vi "Create Review Test.vi"() -> ()   [LabVIEW 2018, in "Collaborator.lvlib"]
uses:
  Collaborator.lvlib
  Command Configuration.ctl
  Web Client/Web Client.lvclass
  <vilib>/JDP Science/JSONtext/JSONtext.lvlib
panel:
  out "error out":errorcluster
  out "Response":string
  in  "Address":string
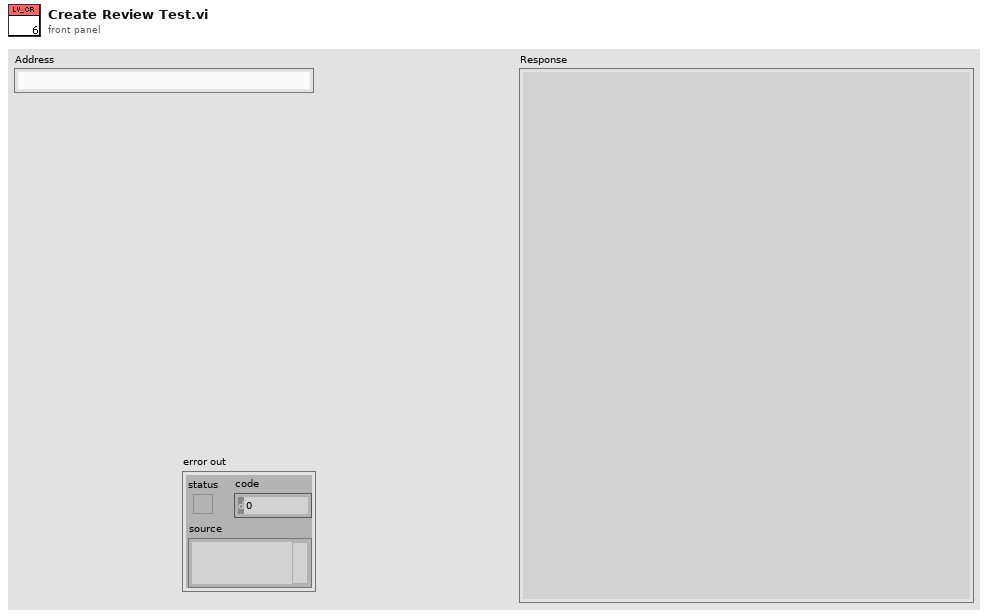
[diagram p1: front panel]
types:
  T1 = typedef "Collaborator.lvlib/Command Configuration.ctl" = cluster{"Interface Name":string, "Method Name":string, "Arguments":cluster{"Argument Name":string, "Argument Value":string}[]}
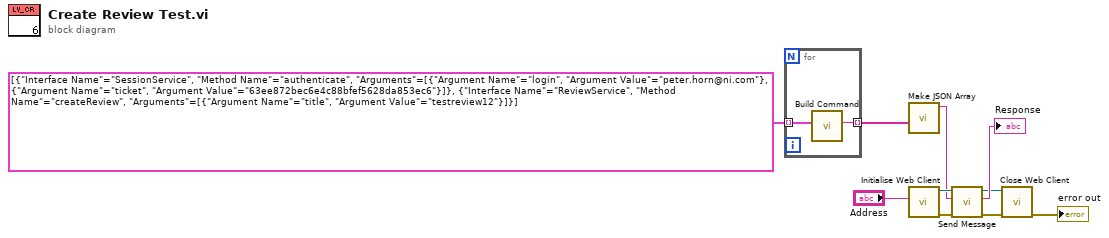
[diagram p0: block diagram]
diagram:
  n1 = for {
    tunnel: [w12] -> w2 mode=indexing
    tunnel: T1[] [{"Interface Name"="SessionService", "Method Name"="authenticate", "Arguments"=[{"Argument Name"="login", "Argument Value"="peter.horn@ni.com"}, {"Argument Name"="ticket", "Argument Value"="63ee872bec6e4c88bfef5628da853ec6"}]}, {"Interface Name"="ReviewService", "Method Name"="createReview", "Arguments"=[{"Argument Name"="title", "Argument Value"="testreview12"}]}] ("Array") -> [w11] mode=indexing
    n2 = call "Build Command.vi"("Command Definition"=w11) -> ("Command"=w12:string)  [unwired: 10 in]
  }
  n3 = call <vilib>:"Make JSON Array.vi"("JSON Elements"=w2) -> ("<JSON>"=w1:string)  [unwired: 9 in, 1 out]
  n4 = call "Initialise Web Client.vi"("Address"="Address") -> ("error out"=w9:errorcluster, "Web Client out"=w10:refnum<class "Web Client.lvclass">)  [unwired: 9 in]
  n5 = call "Send Message.vi"("error in (no error)"=w9, "Message Data"=w1, "Web Client in"=w10) -> ("error out"=w8:errorcluster, "Response"=→"Response":string, "Web Client out"=w4:refnum<class "Web Client.lvclass">)  [unwired: 6 in]
  n6 = call "Close Web Client.vi"("error in (no error)"=w8, "Web Client in"=w4) -> ("error out"=→"error out":errorcluster)  [unwired: 9 in]
